vi "Set State (FGV).vi"(8 "Error In":errorcluster, 10 "Action":T3, 11 "State Input":T2) -> (0 "Error Out":errorcluster, 2 "Controller Output":T1, 3 "State Output":T2)   [LabVIEW 2018]
doc: "This VI realizes a functional global variable that either stores or returns the current state of the FSM, and generates the ouput associated with the state."
uses:
  controls/Enum Defining FGV Action.ctl
  controls/Enum Defining FSM State.ctl
  controls/Cluster for displaying  LED outputs.ctl
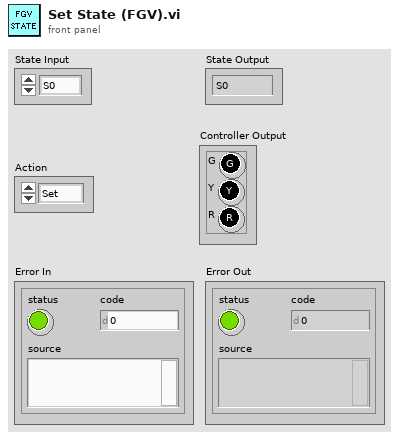
[diagram p1: front panel]
types:
  T1 = typedef "Cluster for displaying  LED outputs.ctl" = cluster{"G":bool, "Y":bool, "R":bool}
  T2 = typedef "Enum Defining FSM State.ctl" = enum16{"S0", "S1", "S2", "S3"}
  T3 = typedef "Enum Defining FGV Action.ctl" = enum16{"Set", "Get"}
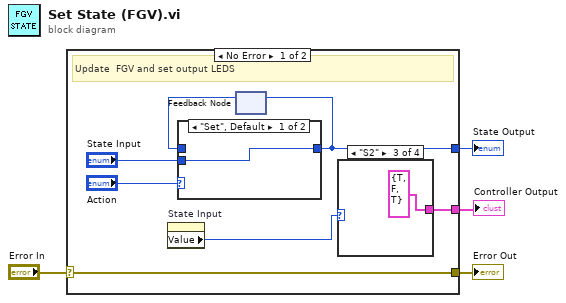
[diagram p0: block diagram]
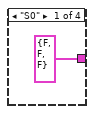
[diagram p2: hidden frame]
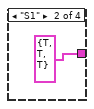
[diagram p3: hidden frame]
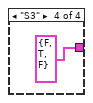
[diagram p4: hidden frame]
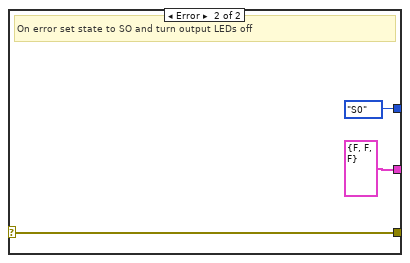
[diagram p6: hidden frame]
diagram:
  n1 = case shown="No Error" "Error In" {
    selector: "Error In" -> [w10 w20]
    tunnel: [w10 w20] -> w3
    tunnel: [w7 Enum_Defining_FSM_State."S0" ("Input State")] -> w2
    tunnel: [w5 T1 {"G"=FALSE, "Y"=FALSE, "R"=FALSE} ("Controller Ouput")] -> w1
    frame No Error {
      # "Update  FGV and set output LEDS"
      n2 = property on="State Input" class="Enum (strict)"() -> ("Value"=w6:T2)  [unwired: 2 in, 2 out]
      n3 = feedback #1() -> (w8:T2)  [unwired: 1 in]
      n4 = case shown="\"Set\", Default" "Action" {
        tunnel: [w16 w17] -> w7
        tunnel: "State Input" -> [w16 _]
        tunnel: w8 -> [_ w17]
        frame "Set", Default {
        }
        frame "Get" {
        }
      }
      n5 = feedback-in #1(w7) -> ()
      n6 = case shown="\"S2\"" w6 {
        tunnel: [T1 {"G"=FALSE, "Y"=FALSE, "R"=FALSE} ("LED Outputs") T1 {"G"=TRUE, "Y"=TRUE, "R"=TRUE} ("LED Outputs") T1 {"G"=TRUE, "Y"=FALSE, "R"=TRUE} ("LED Outputs") T1 {"G"=FALSE, "Y"=TRUE, "R"=FALSE} ("LED Outputs")] -> w5
        frame "S0" {
        }
        frame "S1" {
        }
        frame "S2" {
        }
        frame "S3" {
        }
      }
    }
    frame Error {
      # "On error set state to SO and turn output LEDs off"
    }
  }
  "Error Out" <- w3
  "State Output" <- w2
  "Controller Output" <- w1
